vi "WPVector4 IGVC removal.vi"(6 "WP Vector Input":dbl[](array[numeric]), 7 "Robot Lat and Long":dbl[](array[numeric]), 8 "Num of WPs":dbl, 9 "Heading":dbl, 10 "WP Num Input":dbl, 11 "All WPs Cluster":cluster{"WP Lats":dbl[], "WP Longs":dbl[]}) -> (0 "WP Number":i32, 3 "Angle in degrees and Distance in meters":dbl[](array[numeric]))   [LabVIEW 2014]
panel:
  out "wp num":dbl
  # "Inputs:"
  # "Outputs:"
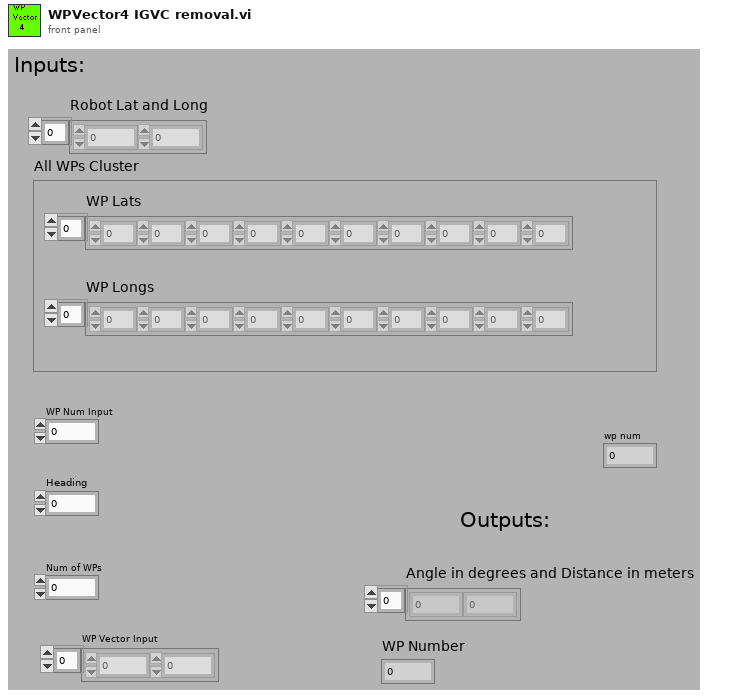
[diagram p1: front panel]
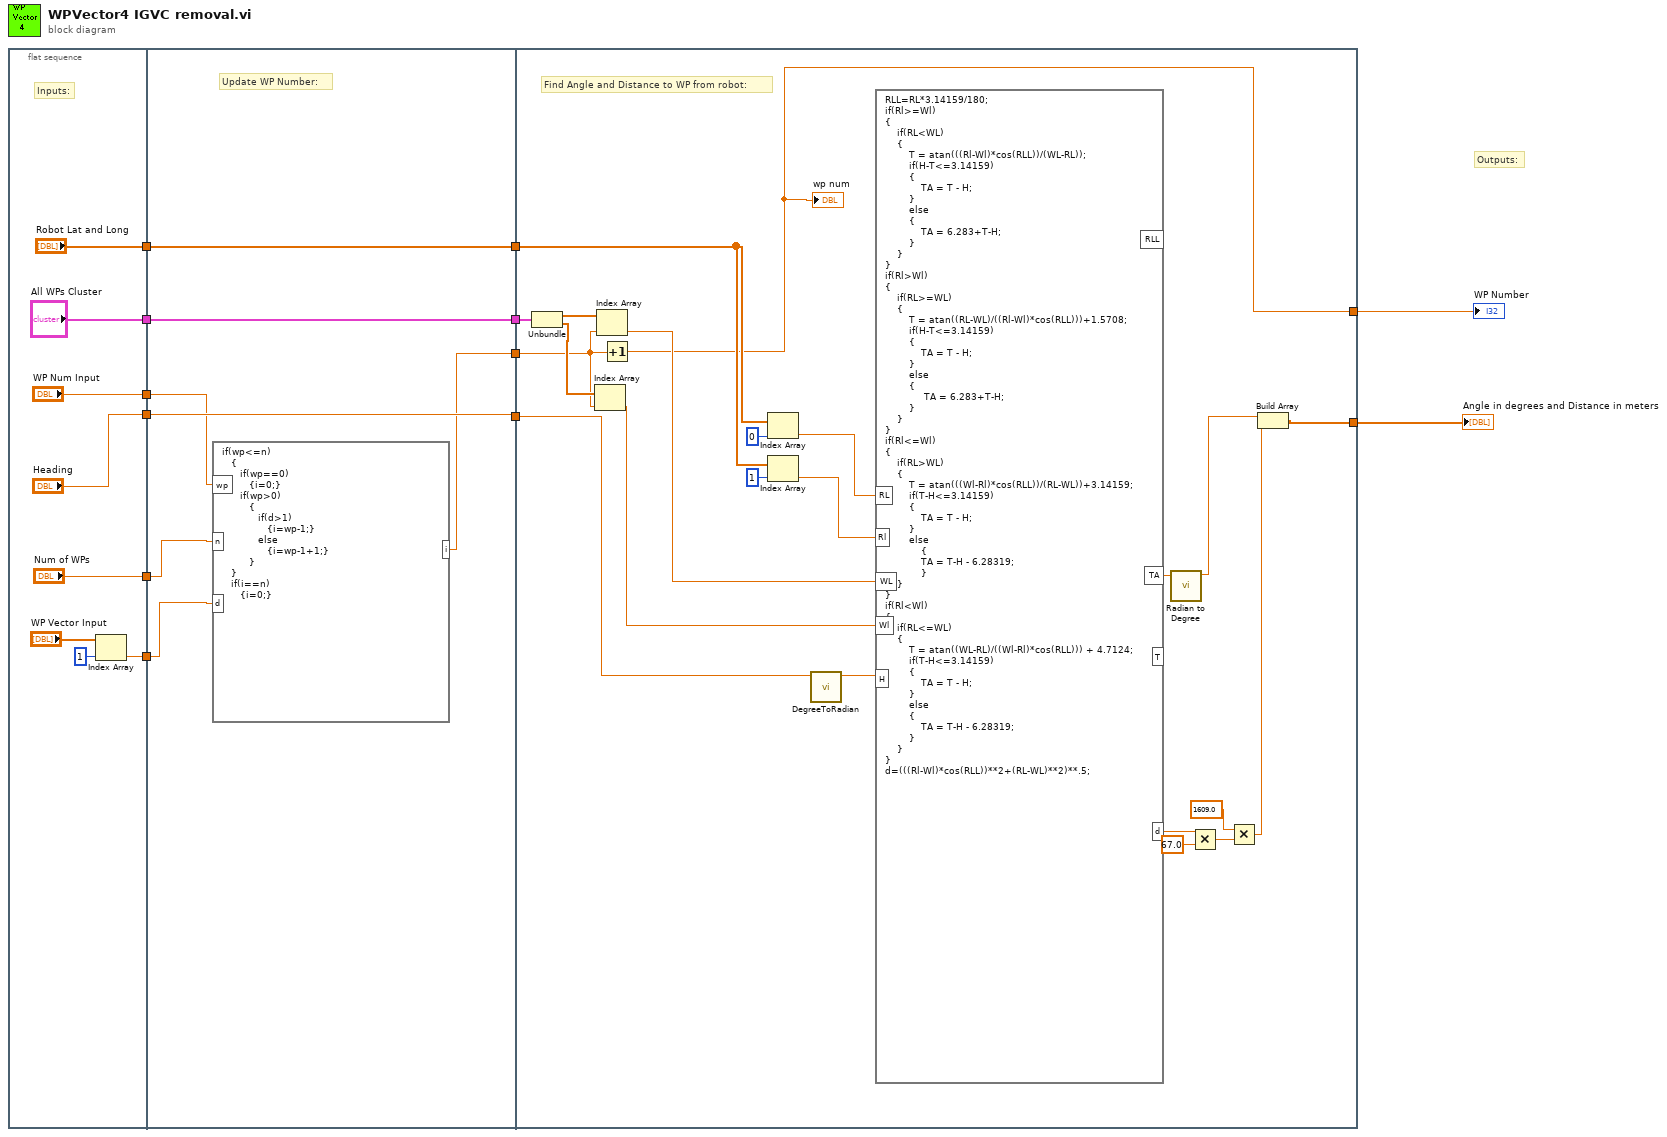
[diagram p0: block diagram]
diagram:
  # "Outputs:"
  n1 = flat-sequence {
    tunnel: ["Heading"] -> w12
    tunnel: ["Robot Lat and Long"] -> w11
    tunnel: ["All WPs Cluster"] -> w10
    tunnel: ["Num of WPs"] -> w3
    tunnel: ["WP Num Input"] -> w2
    tunnel: [w13] -> w1
    tunnel: w12 -> [w25]
    tunnel: w11 -> [w27]
    tunnel: w10 -> [w26]
    tunnel: [w25] -> w9
    tunnel: [w27] -> w8
    tunnel: [w26] -> w7
    tunnel: [w21] -> w6
    tunnel: w3 -> [w22]
    tunnel: w2 -> [w23]
    tunnel: w1 -> [w24]
    tunnel: w9 -> [w35]
    tunnel: w8 -> [w30]
    tunnel: w7 -> [w32]
    tunnel: w6 -> [w31]
    tunnel: [w28] -> w5
    tunnel: [w29] -> w4
    frame #0 {
      # "Inputs:"
      n2 = Index Array(array="WP Vector Input", index=1) -> (element=w13:dbl)
    }
    frame #1 {
      # "Update WP Number:"
      n3 = formula code="if(wp<=n)\n   {\n      if(wp==0)\n         {i=0;}\n      if(wp>0)\n         {\n            if(d>1)\n               {i=wp-1;}\n            else\n               {i=wp-1+1;}\n         }\n   }\n   if(i==n)\n      {i=0;}"("wp"=w23, "n"=w22, "d"=w24) -> ("i"=w21:dbl)
    }
    frame #2 {
      # "Find Angle and Distance to WP from robot:"
      n4 = Unbundle(w32) -> ("WP Lats"=w33:dbl[], "WP Longs"=w48:dbl[])
      n5 = Index Array(array=w48, index=w31) -> (element=w34:dbl)
      n6 = Index Array(array=w33, index=w31) -> (element=w49:dbl)
      n7 = Increment(x=w31) -> (x+1=w28:dbl)
      "wp num" <- w28
      n8 = Index Array(array=w30, index=0) -> (element=w42:dbl)
      n9 = Index Array(array=w30, index=1) -> (element=w45:dbl)
      n10 = call "DegreeToRadian.vi"("Degrees"=w35) -> ("Radians"=w36:dbl)  [unwired: 10 in]
      n11 = formula code="RLL=RL*3.14159/180;\nif(Rl>=Wl)  \n{\n    if(RL<WL)\n    {\n        T = atan(((Rl-Wl)*cos(RLL))/(WL-RL));\n        if(H-T<=3.14159)\n        {\n            TA = T - H;\n        }\n        else \n        {\n            TA = 6.283+T-H;\n        }\n    }\n}\nif(Rl>Wl)\n{\n    if(RL>=WL)\n    {\n        T = atan((RL-WL)/((Rl-Wl)*cos(RLL)))+1.5708;\n        if(H-T<=3.14159)\n        {\n            TA = T - H;\n        }\n        else\n        {\n             TA = 6.283+T-H;\n        }\n    }\n}\nif(Rl<=Wl)\n{\n    if(RL>WL)\n    {\n        T = atan(((Wl-Rl)*cos(RLL))/(RL-WL))+3.14159;\n        if(T-H<=3.14159)\n        {\n            TA = T - H;\n        }\n        else\n            {\n            TA = T-H - 6.28319;\n            }\n    }\n}\nif(Rl<Wl)\n{\n    if(RL<=WL)\n    {\n        T = atan((WL-RL)/((Wl-Rl)*cos(RLL))) + 4.7124;\n        if(T-H<=3.14159)\n        {\n            TA = T - H;\n        }\n        else\n        {\n            TA = T-H - 6.28319;\n        }\n    }\n}\nd=(((Rl-Wl)*cos(RLL))**2+(RL-WL)**2)**.5;"("RL"=w42, "Rl"=w45, "WL"=w49, "Wl"=w34, "H"=w36) -> ("TA"=w37:dbl, "d"=w38:dbl)  [unwired: 2 out]
      n12 = call "Radian to Degree.vi"("Radians"=w37) -> ("Degrees"=w46:dbl)  [unwired: 10 in]
      n13 = Multiply(x=w38, y=67.0) -> (x*y=w40:dbl)
      n14 = Multiply(x=1609.0, y=w40) -> (x*y=w47:dbl)
      n15 = Build Array(w46, w47) -> (w29:dbl[])
    }
  }
  "Angle in degrees and Distance in meters" <- w4
  "WP Number" <- w5
